vi "Coerce to 8-Bit Data Type.vi"(0 "image pixel data region in":refnum<data-value>, 5 "image bytes in":u32, 7 "data type in":T1, 11 "error in (no error)":errorcluster) -> (4 "image pixel data region out":refnum<data-value>, 6 "image bytes out":u32, 8 "data type out":T1, 15 "error out":errorcluster)   [LabVIEW 2023, in "GettingStarted_Common_148X_Host.lvlib"]
uses:
  GettingStarted_Common_148X_Host.lvlib
  <instrlib>/FlexRIO/CSI-2/v2/Common/Types/LLP Data Type.ctl
  <instrlib>/FlexRIO/CSI-2/v2/Common/NI CSI-2 API Common v2.lvlib
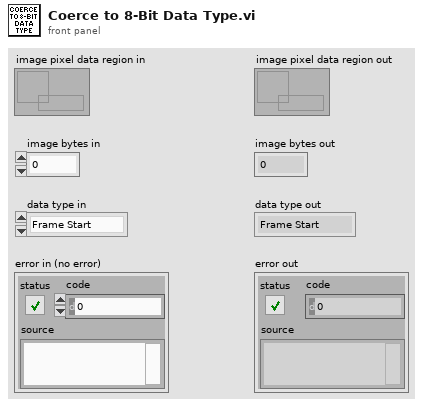
[diagram p1: front panel]
types:
  T1 = typedef "NI CSI-2 API Common v2.lvlib/LLP Data Type.ctl" = enum8{"Frame Start", "Frame End", "Line Start", "Line End", "End of Transmission", "Reserved 0", "Reserved 1", "Reserved 2", "Generic Short Packet 1", "Generic Short Packet 2", "Generic Short Packet 3", "Generic Short Packet 4", "Generic Short Packet 5", "Generic Short Packet 6", "Generic Short Packet 7", "Generic Short Packet 8", "Null", "Blanking Data", "Embedded 8-bit non Image Data", "Generic Long Packet 1", "Generic Long Packet 2", "Generic Long Packet 3", "Generic Long Packet 4", "Reserved 3", "YUV420 8-bit", "YUV420 10-bit", "Legacy YUV420 8-bit", "Reserved 4", "YUV420 8-bit Chroma Shifted", "YUV420 10-bit Chroma Shifted", "YUV422 8-bit", "YUV422 10-bit", "RGB444", "RGB555", "RGB565", "RGB666", "RGB888", "Reserved 5", "Reserved 6", "RAW 24", "RAW 6", "RAW 7", "RAW 8", "RAW 10", "RAW 12", "RAW 14", "RAW 16", "RAW 20", "User Defined 8-bit Data 1", "User Defined 8-bit Data 2", "User Defined 8-bit Data 3", "User Defined 8-bit Data 4", "User Defined 8-bit Data 5", "User Defined 8-bit Data 6", "User Defined 8-bit Data 7", "User Defined 8-bit Data 8", "USL Command", "Reserved 7", "Reserved 8", "Reserved 9", "Reserved 10", "Reserved 11", "Reserved 12", "LRTE EPD Spacer"}
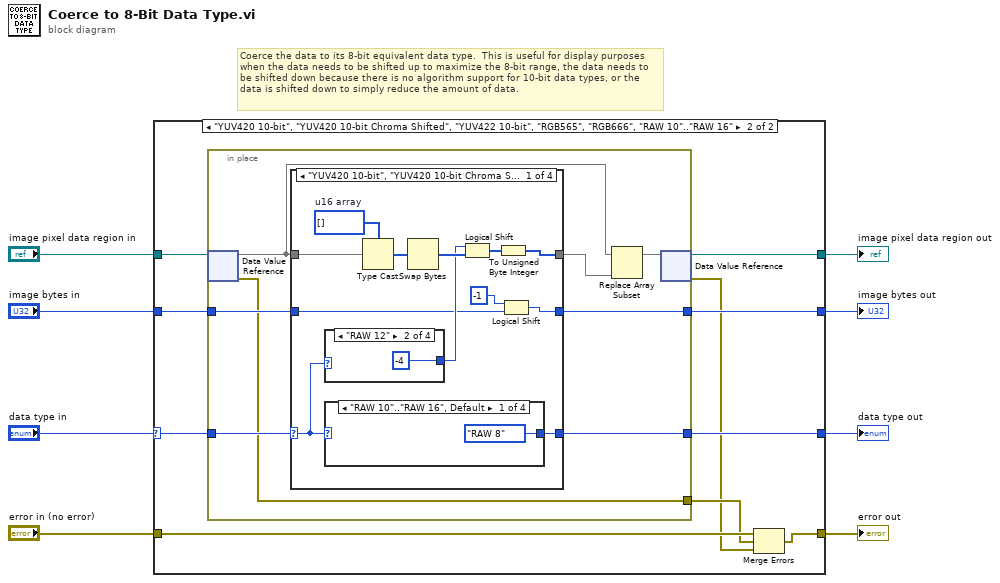
[diagram p0: block diagram]
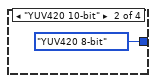
[diagram p3: hidden frame]
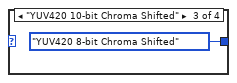
[diagram p4: hidden frame]
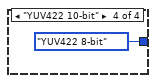
[diagram p5: hidden frame]
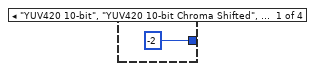
[diagram p6: hidden frame]
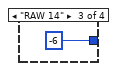
[diagram p7: hidden frame]
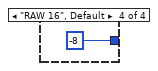
[diagram p8: hidden frame]
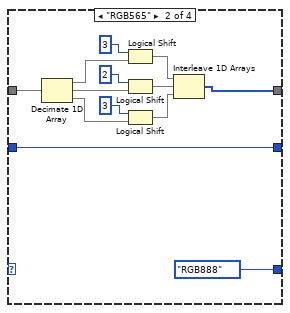
[diagram p9: hidden frame]
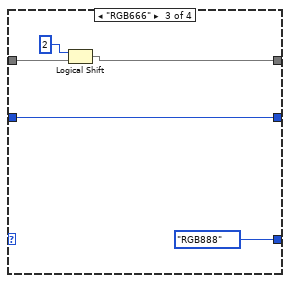
[diagram p10: hidden frame]
diagram:
  # "Coerce the data to its 8-bit equivalent data type.  This is useful for display purposes when the data needs to be shifted up to maximize the 8-bit range, the data needs to be shifted down because there is no algorithm support for 10-bit data types, or the data is shifted down to simply reduce the amount of data."
  n1 = case shown="\"YUV420 10-bit\", \"YUV420 10-bit Chroma Shifted\", \"YUV422 10-bit\", \"RGB565\", \"RGB666\", \"RAW 10\"..\"RAW 16\"" "data type in" {
    selector: "data type in" -> [w11 w20]
    tunnel: "image pixel data region in" -> [w12 w22]
    tunnel: [w11 w21] -> w7
    tunnel: [w10 w19] -> w5
    tunnel: "image bytes in" -> [w10 w18]
    tunnel: [w12 w17] -> w3
    tunnel: "error in (no error)" -> [w9 w16]
    tunnel: [w9 w13] -> w1
    frame Default {
    }
    frame "YUV420 10-bit", "YUV420 10-bit Chroma Shifted", "YUV422 10-bit", "RGB565", "RGB666", "RAW 10".."RAW 16" {
      n2 = in-place {
        in-place-border: w20 -> [w30]
        in-place-border: [w29] -> w21
        in-place-border: [w28] -> w19
        in-place-border: w18 -> [w27]
        in-place-border: [w26] -> w15
        n3 = in-place-dvr #1(w22) -> (w25:u8[], w26:errorcluster)
        n4 = case shown="\"YUV420 10-bit\", \"YUV420 10-bit Chroma Shifted\", \"YUV422 10-bit\", \"RAW 10\"..\"RAW 16\"" w30 {
          selector: w30 -> [w31 _ _ w69]
          tunnel: w25 -> [w37 w63 w68 w71]
          tunnel: [w36 w52 w66 w71] -> w24
          tunnel: [w42 LLP_Data_Type."RGB888" ("data type in") LLP_Data_Type."RGB888" ("data type in") w69] -> w29
          tunnel: [w32 w59 w64 w70] -> w28
          tunnel: w27 -> [w34 w59 w64 w70]
          frame "YUV420 10-bit", "YUV420 10-bit Chroma Shifted", "YUV422 10-bit", "RAW 10".."RAW 16" {
            w41 = u16[] []  # u16 array
            n5 = case shown="\"RAW 12\"" w31 {
              tunnel: [i16 -2 ("y") i16 -4 ("y") i16 -6 ("y") i16 -8 ("y")] -> w35
              frame "YUV420 10-bit", "YUV420 10-bit Chroma Shifted", "YUV422 10-bit", "RAW 10" {
              }
              frame "RAW 12" {
              }
              frame "RAW 14" {
              }
              frame "RAW 16", Default {
              }
            }
            n6 = case shown="\"RAW 10\"..\"RAW 16\", Default" w31 {
              tunnel: [LLP_Data_Type."RAW 8" ("data type in") LLP_Data_Type."YUV420 8-bit" ("data type in") LLP_Data_Type."YUV420 8-bit Chroma Shifted" ("data type in") LLP_Data_Type."YUV422 8-bit" ("data type in")] -> w42
              frame "RAW 10".."RAW 16", Default {
              }
              frame "YUV420 10-bit" {
              }
              frame "YUV420 10-bit Chroma Shifted" {
              }
              frame "YUV422 10-bit" {
              }
            }
            n7 = Type Cast(type=w41, x=w37) -> (*(type *) &x=w40:u16[])
            n8 = Swap Bytes(anything=w40) -> (byte swapped=w39:u16[])
            n9 = Logical Shift(y=w35, x=w39) -> (x << y=w38:u16[])
            n10 = To Unsigned Byte Integer(number=w38) -> (unsigned 8bit integer=w36:u8[])
            n11 = Logical Shift(y=i16 -1, x=w34) -> (x << y=w32:u32)
          }
          frame "RGB565" {
            n12 = Decimate 1D Array(w63) -> (w58:u8[], w54:u8[], w53:u8[])
            n13 = Logical Shift(y=i16 3, x=w58) -> (x << y=w55:u8[])
            n14 = Logical Shift(y=i16 2, x=w54) -> (x << y=w56:u8[])
            n15 = Logical Shift(y=i16 3, x=w53) -> (x << y=w57:u8[])
            n16 = Interleave 1D Arrays(w55, w56, w57) -> (w52:u8[])
          }
          frame "RGB666" {
            n17 = Logical Shift(y=i16 2, x=w68) -> (x << y=w66:u8[])
          }
          frame Default {
          }
        }
        n18 = Replace Array Subset(array=w25, new element=w24) -> (w23:u8[])  [unwired: 1 in]
        n19 = in-place-dvr #1(w23) -> (w17:refnum<data-value>, w14:errorcluster)
      }
      n20 = Merge Errors(w16, w15, w14) -> (w13:errorcluster)
    }
  }
  "error out" <- w1
  "data type out" <- w7
  "image pixel data region out" <- w3
  "image bytes out" <- w5
